vi "Classify Error.vi"(10 "Error Code":i32) -> (2 "Error Classification":i32)   [LabVIEW 2015, in "Tektronix DPO MSO 2000 4000 Series.lvlib"]
doc: "This VI takes error codes and returns whether it is an error, warning, or to be ignored."
uses:
  Tektronix DPO MSO 2000 4000 Series.lvlib
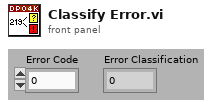
[diagram p1: front panel]
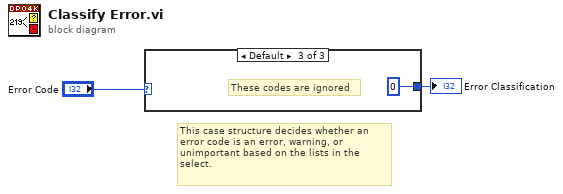
[diagram p0: block diagram]
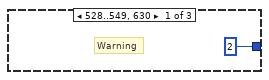
[diagram p2: hidden frame]
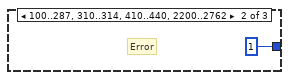
[diagram p3: hidden frame]
diagram:
  # "This case structure decides whether an error code is an error, warning, or unimportant based on the lists in the select."
  n1 = case shown="Default" "Error Code" {
    tunnel: [2 1 0] -> w1
    frame 528..549, 630 {
      # "Warning"
    }
    frame 100..287, 310..314, 410..440, 2200..2762 {
      # "Error"
    }
    frame Default {
      # "These codes are ignored"
    }
  }
  "Error Classification" <- w1
